vi "Analytics update.vi"(8 "error in (no error)":errorcluster, 9 "SM Enqueuer":refnum<class "Message Enqueuer.lvclass">, 10 "User Interface enqueuer":refnum<class "Message Enqueuer.lvclass">, 11 "analyticsButtonState":bool) -> (0 "error out":errorcluster)   [LabVIEW 2019, in "ZenGage v3.0 UI.lvclass"]
uses:
  ZenGage v3.0 UI.lvclass
  User Interface Messages/User Interface messages/Call function_UI Msg/ButtonPress_UI.lvclass
  Type Definitions/General/Output choice.ctl
  <vilib>/ActorFramework/Message Enqueuer/Message Enqueuer.lvclass
  Common/Controls/Acknowledgement.ctl
  Type Definitions/General/OutputDetails.ctl
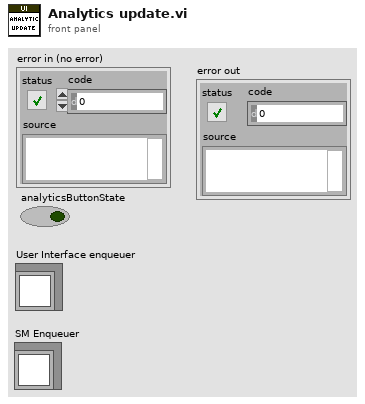
[diagram p1: front panel]
types:
  T1 = typedef "ZenGage v3.0 UI.lvclass/OutputDetails.ctl" = cluster{"Acknowledgement_SM":T2, "Button name":string, "PartDetails":cluster{"PartName":string, "ConnectorsInReel":u64, "TotalCounts":u64, "OperatorName":string, "StampingMachineID":u32}, "SensorName":string, "CameraName":string, "PopupFeedbackDetails":cluster{"Pop-up Type":enum16{"Open Logo Display", "Close Logo Display", "Open Loading Bar", "Close Loading Bar", "Open Alert Display", "Close Alert Display", "One button dialog box", "Two button dialog box", "User Authentication"}, "Message":string, "Pressed Button":string}, "EventResponse":string, "ErrorMessage":string, "FailCountIgnore":cluster{"ReelIgnoreCount":u64, "ProductionIgnoreCount":u64}}
  T2 = typedef "Acknowledgement.ctl" = cluster{"Enqueuer":refnum<class "Message Enqueuer.lvclass">, "VIReference":refnum<vi>, "VIName":string}
  T3 = typedef "ZenGage v3.0 UI.lvclass/Output choice.ctl" = enum16{"SendIgnoredFailCount", "SendPartDetails", "ButtonPress", "SendAcknowledgement", "InitiateCameraDiagnostics", "InitiateSensorDiagnostics", "SendPopupResponse", "SendEventReasonResponse", "SendErrorDetails"}
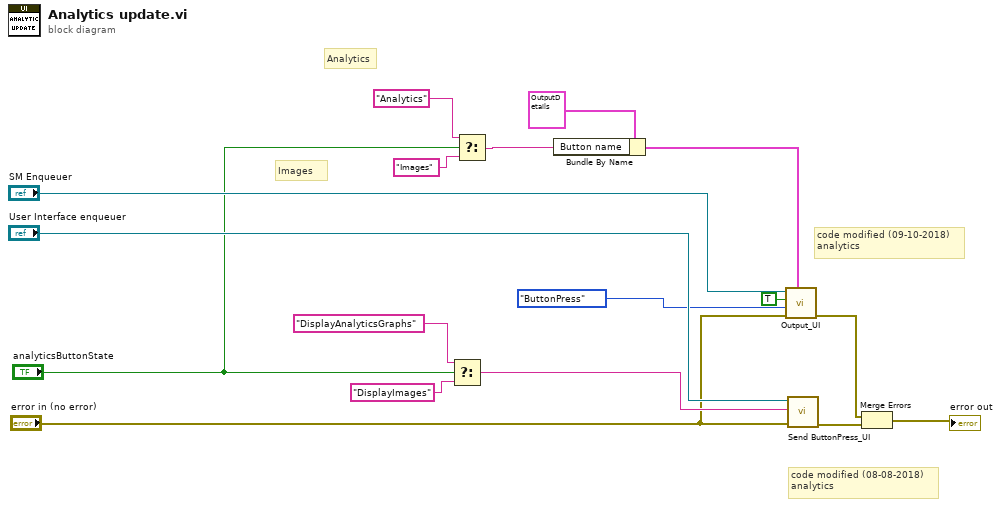
[diagram p0: block diagram]
diagram:
  # "Images"
  # "Analytics"
  # "code modified (09-10-2018)\nanalytics"
  # "code modified (08-08-2018)\nanalytics"
  n1 = Select(t="DisplayAnalyticsGraphs" ("FunctionalityName"), s="analyticsButtonState", f="DisplayImages" ("FunctionalityName")) -> (s? t:f=w14:string)
  n2 = Select(t="Analytics" ("FunctionalityName"), s="analyticsButtonState", f="Images" ("FunctionalityName")) -> (s? t:f=w5:string)
  n3 = Bundle By Name(cluster=T1 {"Acknowledgement_SM"={"Enqueuer"=refnum, "VIReference"=refnum, "VIName"=""}, "Button name"="", "PartDetails"={"PartName"="", "ConnectorsInReel"=0, "TotalCounts"=0, "OperatorName"="", "StampingMachineID"=0}, "SensorName"="", "CameraName"="", "PopupFeedbackDetails"={"Pop-up Type"=enum."Open Logo Display", "Message"="", "Pressed Button"=""}, "EventResponse"="", "ErrorMessage"="", "FailCountIgnore"={"ReelIgnoreCount"=0, "ProductionIgnoreCount"=0}} ("OutputDetails"), "Button name"=w5) -> (w4:T1)
  n4 = call "Output_UI.vi"("OutputDetails"=w4, "error in"="error in (no error)", "Functionality"=Output_choice."ButtonPress", "Testbench"=TRUE, "SMEnqueuer"="SM Enqueuer") -> ("error out"=w1:errorcluster)  [unwired: 6 in]
  n5 = call "Send ButtonPress_UI.vi"("error in (no error)"="error in (no error)", "FunctionalityName"=w14, "Message Enqueuer"="User Interface enqueuer") -> ("error out"=w3:errorcluster)  [unwired: 7 in, 1 out]
  n6 = Merge Errors(w1, w3) -> (→"error out":errorcluster)
